vi "OEE_SCREEN_2.vi"(8 "error_in":errorcluster, 11 "all_config_info":T2={"main_ini_file"={"SQL Driver"="", "SQL Server"="", "SQL Database"="", "SQL UID"="", "Reference table"="", "Reference history"="", "Archivisation CFG table"="", "Archivisation CFG history"="", "User table"="", "User history"="", "Default reference"="", "Update pulse[ms]"=0, "default language"="", "SCREEN 1 Left"=0, "SCREEN 1 Top"=10, "SCREEN 1 Width"=0, "SCREEN 1 Height"=0, "SCREEN 2 Left"=0, "SCREEN 2 Top"=0, "SCREEN 2 Width"=0, "SCREEN 2 Height"=10}, "SQL Password"="", "queue_refnums"={"MAIN_queue"=refnum, "SCREEN_1_queue"=refnum, "SCREEN_2_queue"=refnum, "PULSE_queue"=refnum, "GRAPH_TOGGLE_queue"=refnum}}) -> (0 "error_out":errorcluster)   [LabVIEW 2020]
uses:
  ini/typedef/OEE_all_config_info.ctl
  ini/typedef/OEE_main_ini_file.ctl
  queues/typedef/OEE_queue_refnums.ctl
  queues/typedef/OEE_MAIN_queue_element.ctl
  MAIN/OEE_MAIN_sequence_state.ctl
  queues/typedef/OEE_SCREEN_1_queue_element.ctl
  SCREEN_1/OEE_SCREEN_1_sequence_state.ctl
  queues/typedef/OEE_SCREEN_2_queue_element.ctl
  OEE_SCREEN_2_sequence_state.ctl
  queues/typedef/OEE_PULSE_queue_element.ctl
  PULSE/OEE_PULSE_sequence_state.ctl
  queues/typedef/OEE_GRAPH_TOGGLE_TIMER_queue_element.ctl
  GRAPH_TOGGLE_TIMER/OEE_GRAPH_TOGGLE_TIMER_sequence_state.ctl
  typedef/SCREEN_2.ctl
  <vilib>/Utility/miscctls.llb/LVRectTypeDef.ctl
  FGV/FGV_SCREEN_2_graph_accumulative/FGV_SCREEN_2_graph_accumulative.ctl
  FGV/FGV_SCREEN_2_graph_accumulative/FGV_SCREEN_2_graph_accumulative_references.ctl
  FGV/FGV_SCREEN_2_graph_hourly/FGV_SCREEN_2_graph_hourly.ctl
  FGV/FGV_SCREEN_2_graph_hourly/FGV_SCREEN_2_graph_hourly_references.ctl
  <vilib>/Utility/error.llb/DialogType.ctl
  _misc/AULocalize/SubVIs/RegisterVI.vi
  _misc/AULocalize/SubVIs/Get Localized Phrase Compact Interface 0D.vi
panel:
  out "labels_picture_hourly":picture
  out "graph_hourly":cluster{dbl[], dbl[]}[](graph) caption="ПОЧАСОВАЯ ЦЕЛЬ VS АКТУАЛЬНЫЕ ЗНАЧЕНИЯ"
  out "labels_picture_accumulative":picture
  out "graph_accumulative":cluster{dbl[], dbl[]}[](graph) caption="НАКОПИТЕЛЬНАЯ ЦЕЛЬ VS АКТУАЛЬНЫЕ ЗНАЧЕНИЯ"
  out "SCREEN_2":T1={"header_part_no"="-", "header_customer"="-", "performance_percentage"="-", "performance_target"="-", "performance_actual"="-", "performance_header"="PERFORMANCE", "performance_target_header"="TARGET", "performance_actual_header"="ACTUAL", "screen_2_header"=""}
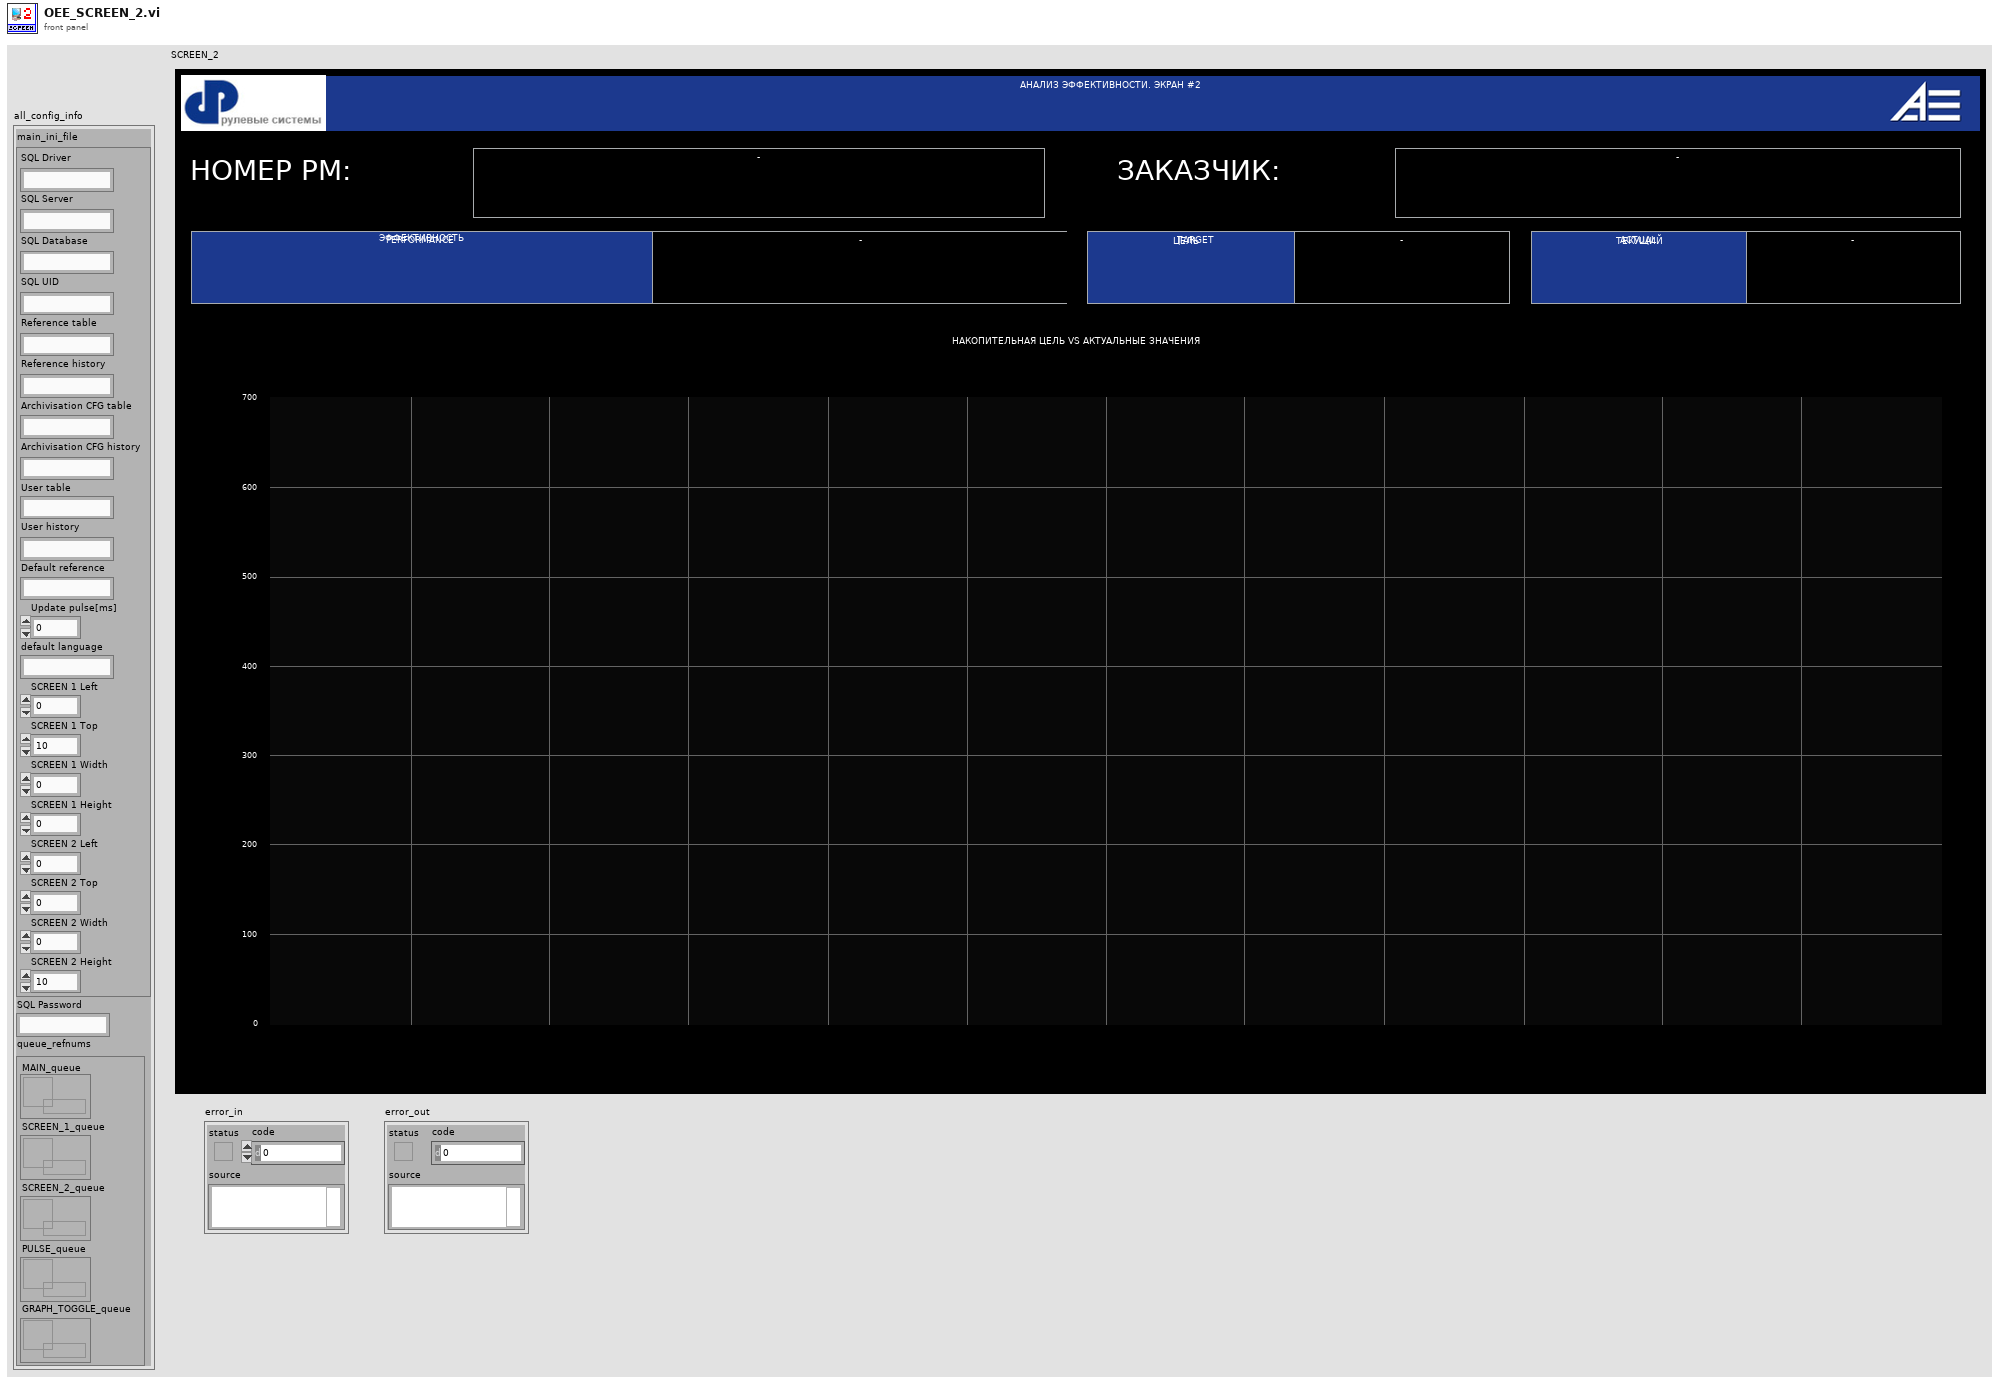
[diagram p1: front panel]
types:
  T1 = typedef "SCREEN_2.ctl" = cluster{"header_part_no":string, "header_customer":string, "performance_percentage":string, "performance_target":string, "performance_actual":string, "performance_header":string, "performance_target_header":string, "performance_actual_header":string, "screen_2_header":string}
  T2 = typedef "OEE_all_config_info.ctl" = cluster{"main_ini_file":T3, "SQL Password":string, "queue_refnums":T4}
  T3 = typedef "OEE_main_ini_file.ctl" = cluster{"SQL Driver":string, "SQL Server":string, "SQL Database":string, "SQL UID":string, "Reference table":string, "Reference history":string, "Archivisation CFG table":string, "Archivisation CFG history":string, "User table":string, "User history":string, "Default reference":string, "Update pulse[ms]":i32, "default language":string, "SCREEN 1 Left":i16, "SCREEN 1 Top":i16, "SCREEN 1 Width":i16, "SCREEN 1 Height":i16, "SCREEN 2 Left":i16, "SCREEN 2 Top":i16, "SCREEN 2 Width":i16, "SCREEN 2 Height":i16}
  T4 = typedef "OEE_queue_refnums.ctl" = cluster{"MAIN_queue":refnum<queue>, "SCREEN_1_queue":refnum<queue>, "SCREEN_2_queue":refnum<queue>, "PULSE_queue":refnum<queue>, "GRAPH_TOGGLE_queue":refnum<queue>}
  T5 = typedef "FGV_SCREEN_2_graph_hourly_references.ctl" = cluster{"graph_hourly":refnum<vi>, "labels_picture_hourly":refnum<vi>, "front_panel_reference":refnum<vi>}
  T6 = typedef "FGV_SCREEN_2_graph_hourly.ctl" = enum16{"initialize", "set_hour_start", "set_hour_end", "set_target", "set_actual", "toggle_visibility", "display"}
  T7 = typedef "FGV_SCREEN_2_graph_accumulative_references.ctl" = cluster{"graph_accumulative":refnum<vi>, "labels_picture_accumulative":refnum<vi>, "front_panel_reference":refnum<vi>}
  T8 = typedef "FGV_SCREEN_2_graph_accumulative.ctl" = enum16{"initialize", "set_hour_start", "set_hour_end", "set_target", "set_actual", "display"}
  T9 = typedef "LVRectTypeDef.ctl" = cluster{"Left":i16, "Top":i16, "Right":i16, "Bottom":i16}
  T10 = typedef "OEE_SCREEN_2_sequence_state.ctl" = enum16{"initialize", "get_next_state", "update", "show", "hide", "error", "stop"}
  T11 = typedef "OEE_GRAPH_TOGGLE_TIMER_sequence_state.ctl" = enum16{"initialize", "get_next_state", "start_toggling", "stop_toggling", "do_toggle", "error", "stop"}
  T12 = typedef "OEE_GRAPH_TOGGLE_TIMER_queue_element.ctl" = cluster{"state":T11, "variable":variant}
  T13 = typedef "OEE_SCREEN_2_queue_element.ctl" = cluster{"state":T10, "variable":variant}
  T14 = typedef "DialogType.ctl" = u16
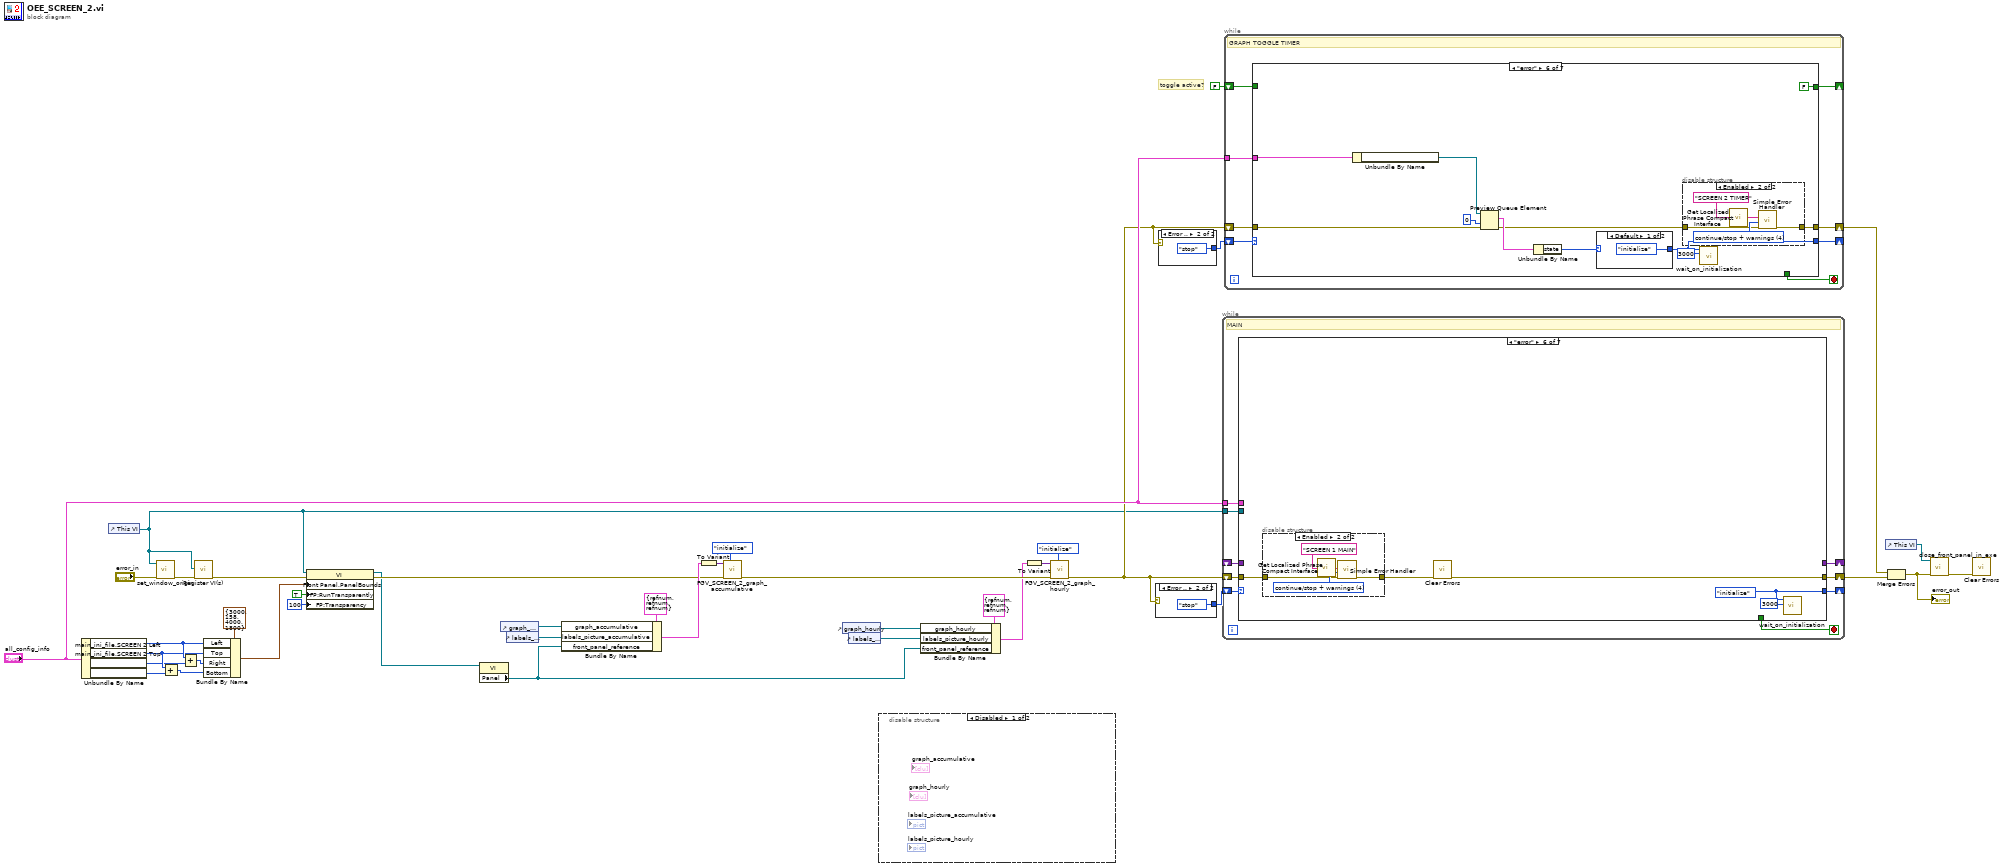
[diagram p0: block diagram]
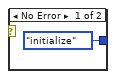
[diagram p2: hidden frame]
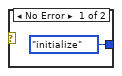
[diagram p3: hidden frame]
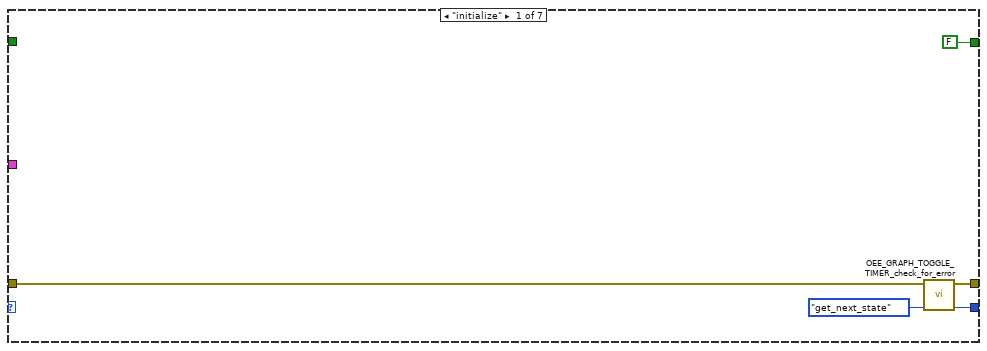
[diagram p4: hidden frame]
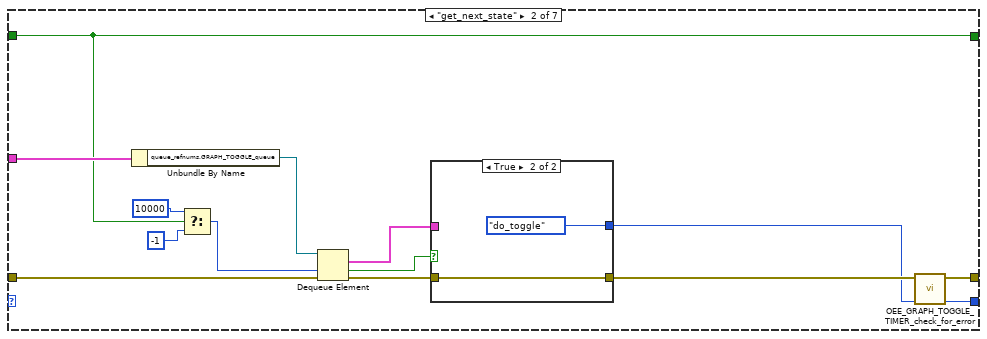
[diagram p5: hidden frame]
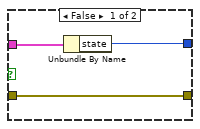
[diagram p6: hidden frame]
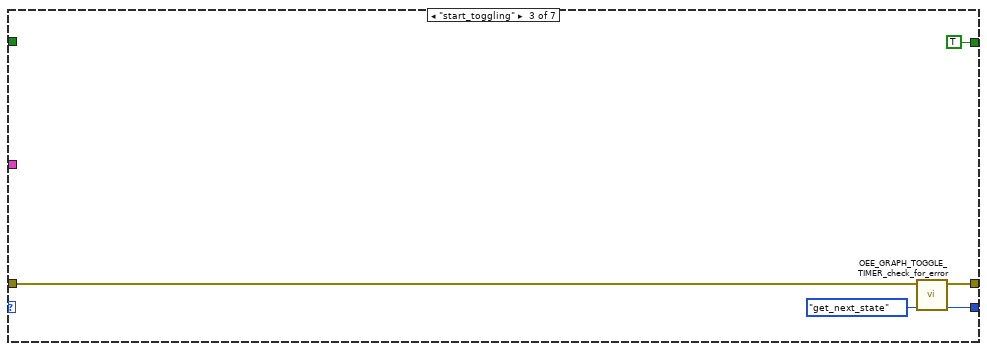
[diagram p7: hidden frame]
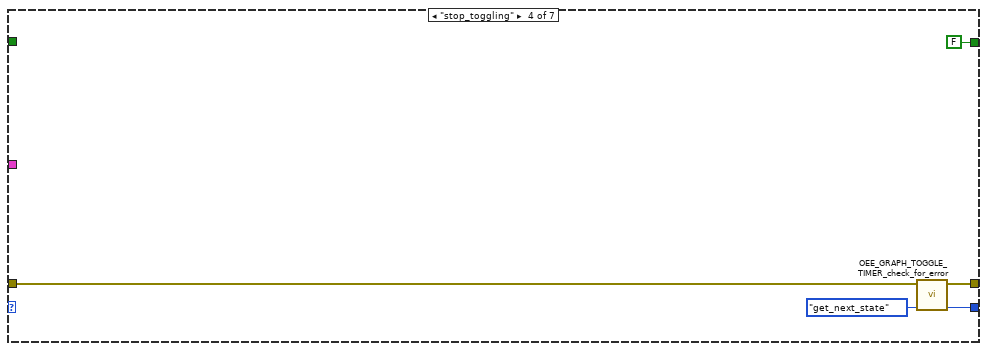
[diagram p8: hidden frame]
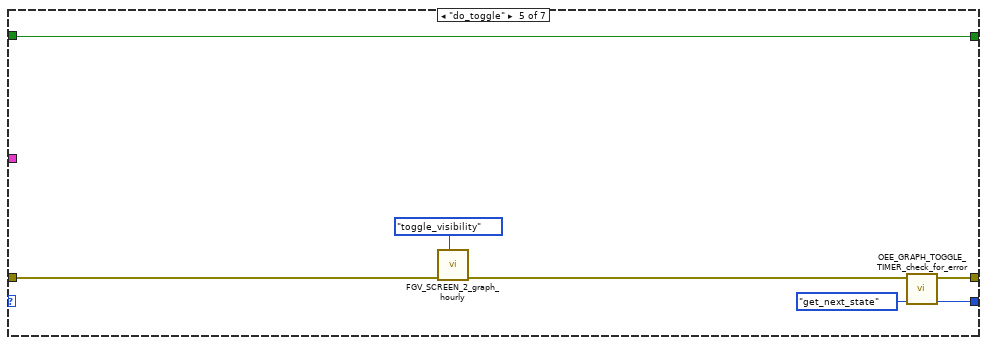
[diagram p9: hidden frame]
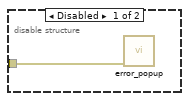
[diagram p10: hidden frame]
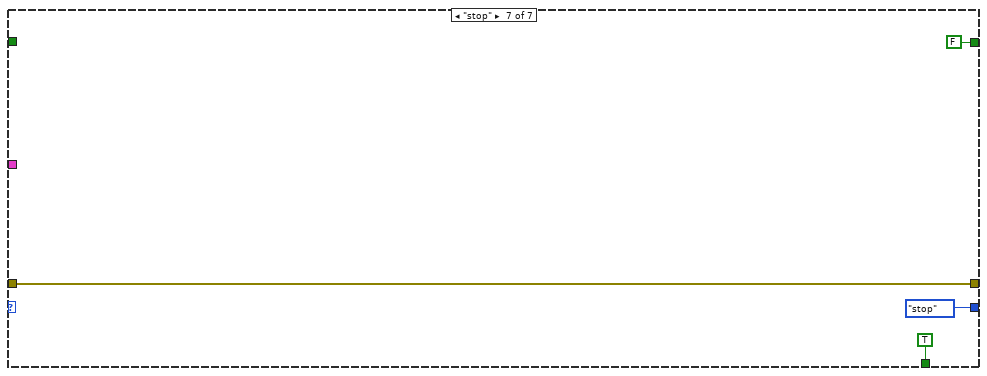
[diagram p12: hidden frame]
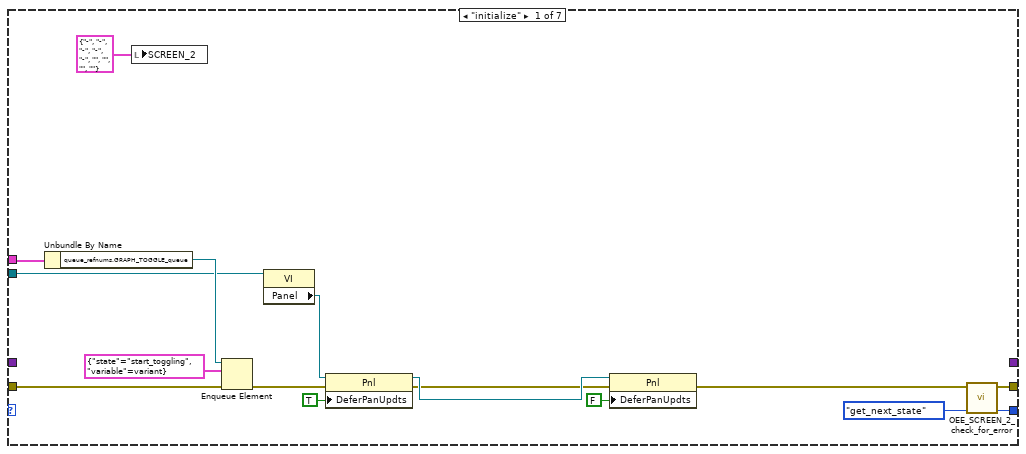
[diagram p14: hidden frame]
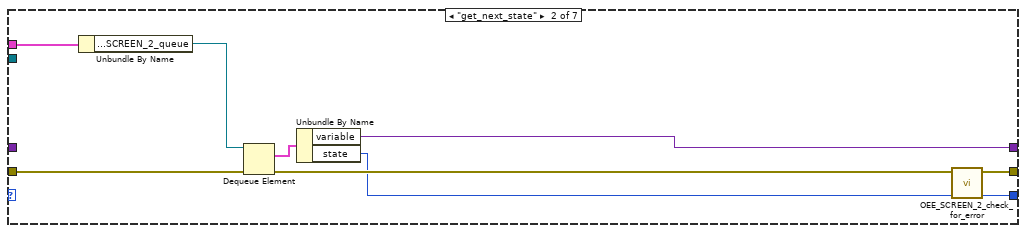
[diagram p15: hidden frame]
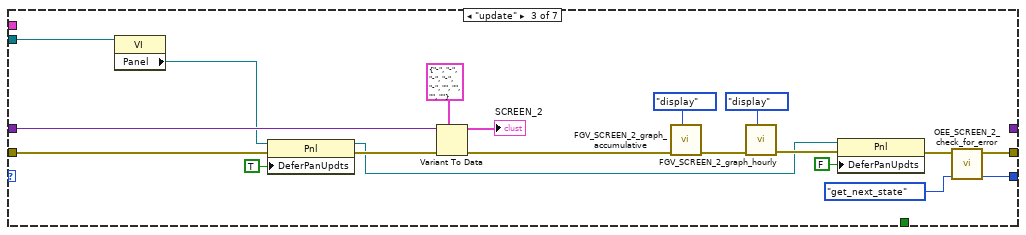
[diagram p16: hidden frame]
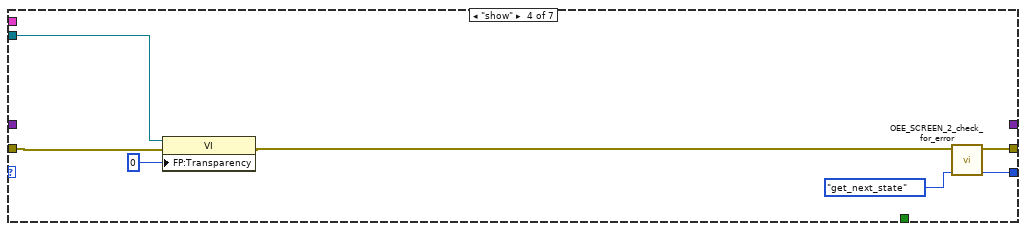
[diagram p17: hidden frame]
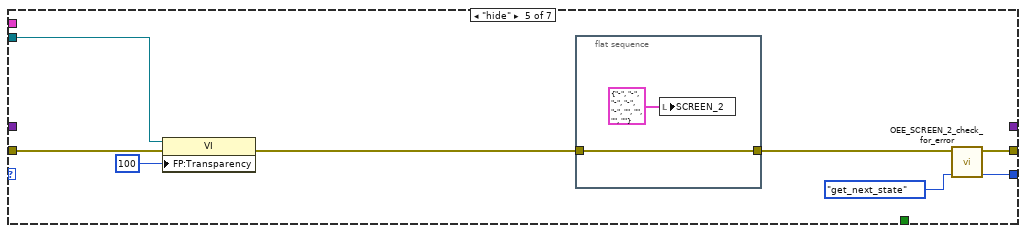
[diagram p18: hidden frame]
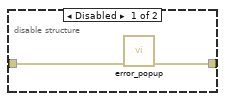
[diagram p19: hidden frame]
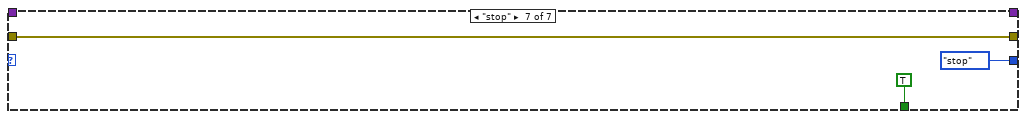
[diagram p20: hidden frame]
diagram:
  # "toggle active?"
  n1 = Unbundle By Name("all_config_info") -> ("main_ini_file.SCREEN 2 Left"=w36:i16, "main_ini_file.SCREEN 2 Top"=w35:i16, "main_ini_file.SCREEN 2 Width"=w34:i16, "main_ini_file.SCREEN 2 Height"=w33:i16)
  n2 = control-ref of="This VI"() -> (w1:refnum<vi>)
  n3 = call "set_window_origin.vi"("error_in"="error_in", "this_vi_reference"=w1) -> ("error_out"=w3:errorcluster)  [unwired: 9 in]
  n4 = Add(x=w35, y=w33) -> (x+y=w38:i16)
  n5 = Add(x=w36, y=w34) -> (x+y=w39:i16)
  n6 = call-poly "Register VI(s).vi"("error in"=w3, "VI Ref"=w1) -> ("error out"=w2:errorcluster)  [unwired: 8 in, 1 out]
  n7 = Bundle By Name(cluster=T9 {"Left"=3000, "Top"=158, "Right"=4000, "Bottom"=1800} ("Front Panel Window:Panel Bounds"), "Left"=w36, "Top"=w35, "Right"=w39, "Bottom"=w38) -> (w7:T9)
  n8 = property class="VI"(reference=w1, error in=w2, "Front Panel.PanelBounds"=w7, "FP:RunTransparently"=TRUE ("Front Panel Window:Run VI Transparently"), "FP:Transparency"=u8 100 ("Front Panel Window:Transparency")) -> (reference out=w8:refnum<vi>, error out=w9:errorcluster)
  n9 = property class="VI"(reference=w8) -> ("Panel"=w12:refnum<vi>)  [unwired: 1 in, 2 out]
  n10 = control-ref of="graph_accumulative"() -> (w30:refnum<vi>)
  n11 = control-ref of="labels_picture_accumulative"() -> (w19:refnum<vi>)
  n12 = Bundle By Name(cluster=T7 {"graph_accumulative"=refnum, "labels_picture_accumulative"=refnum, "front_panel_reference"=refnum} ("OBJ_references"), "graph_accumulative"=w30, "labels_picture_accumulative"=w19, "front_panel_reference"=w12) -> (w28:T7)
  n13 = To Variant(anything=w28) -> (Variant=w29:variant)
  n14 = call "FGV_SCREEN_2_graph_accumulative.vi"("options"=FGV_SCREEN_2_graph_accumulative."initialize", "error_in"=w9, "input"=w29) -> ("error_out"=w27:errorcluster)  [unwired: 8 in]
  n15 = control-ref of="graph_hourly"() -> (w22:refnum<vi>)
  n16 = control-ref of="labels_picture_hourly"() -> (w18:refnum<vi>)
  n17 = disable-structure shown="Disabled" {
    frame Disabled {
    }
    frame Enabled {
    }
  }
  n18 = Bundle By Name(cluster=T5 {"graph_hourly"=refnum, "labels_picture_hourly"=refnum, "front_panel_reference"=refnum} ("graph_hourly_references"), "graph_hourly"=w22, "labels_picture_hourly"=w18, "front_panel_reference"=w12) -> (w24:T5)
  n19 = To Variant(anything=w24) -> (Variant=w25:variant)
  n20 = call "FGV_SCREEN_2_graph_hourly.vi"("options"=FGV_SCREEN_2_graph_hourly."initialize", "error_in"=w27, "input"=w25) -> ("error_out"=w4:errorcluster)  [unwired: 8 in]
  n21 = case shown="Error .." w4 {
    tunnel: [OEE_SCREEN_2_sequence_state."initialize" ("state") OEE_SCREEN_2_sequence_state."stop" ("state")] -> w37
    frame No Error {
    }
    frame Error {
    }
  }
  n22 = case shown="Error .." w4 {
    tunnel: [OEE_GRAPH_TOGGLE_TIMER_sequence_state."initialize" ("OBJ_GUI_TIMER_sequence_state") OEE_GRAPH_TOGGLE_TIMER_sequence_state."stop" ("OBJ_GUI_TIMER_sequence_state")] -> w15
    frame No Error {
    }
    frame Error {
    }
  }
  n23 = while {
    shift-right: [w50] -> _
    shift-left: w37 -> [w51]
    shift-right: [w49] -> _
    shift-left: _ -> [w48]
    shift-right: [w52] -> w14
    shift-left: w4 -> [w53]
    tunnel: "all_config_info" -> [w46]
    tunnel: w1 -> [w45]
    stop <- w47 stop-if-true
    # "MAIN"
    n24 = case shown="\"error\"" w51 {
      tunnel: w53 -> [w65 w74 w82 w100 w108 w115 w129]
      tunnel: [w69 w78 w97 w104 w112 w119 w129] -> w52
      tunnel: [w68 w77 w96 w103 w111 w118 OEE_SCREEN_2_sequence_state."stop" ("state")] -> w50
      tunnel: [_ w72 _ _ _ _ _] -> w49
      tunnel: w48 -> [_ _ w89 _ _ _ _]
      tunnel: [_ _ _ _ _ _ TRUE] -> w47
      tunnel: w46 -> [w66 w71 _ _ _ _ _]
      tunnel: w45 -> [w56 _ w81 w99 w107 _ _]
      frame "initialize" {
        n25 = Unbundle By Name(w66) -> ("queue_refnums.GRAPH_TOGGLE_queue"=w64:refnum<queue>)
        n26 = local write "SCREEN_2"(T1 {"header_part_no"="-", "header_customer"="-", "performance_percentage"="-", "performance_target"="-", "performance_actual"="-", "performance_header"="", "performance_target_header"="", "performance_actual_header"="", "screen_2_header"=""} ("SCREEN_2")) -> ()
        n27 = Enqueue Element(queue=w64, element=T12 {"state"=enum."start_toggling", "variable"=variant}, error in (no error)=w65) -> (error out=w59:errorcluster)  [unwired: 1 in, 2 out]
        n28 = property class="VI"(reference=w56) -> ("Panel"=w55:refnum<vi>)  [unwired: 1 in, 2 out]
        n29 = property class="Pnl"(reference=w55, error in=w59, "DeferPanUpdts"=TRUE ("Defer Panel Updates")) -> (reference out=w57:refnum<vi>, error out=w54:errorcluster)
        n30 = property class="Pnl"(reference=w57, error in=w54, "DeferPanUpdts"=FALSE ("Defer Panel Updates")) -> (error out=w58:errorcluster)  [unwired: 1 out]
        n31 = call "OEE_SCREEN_2_check_for_error.vi"("SCREEN_2_loop_state_in"=OEE_SCREEN_2_sequence_state."get_next_state" ("state"), "error_in"=w58) -> ("SCREEN_2_loop_state_out"=w68:T10, "error_out"=w69:errorcluster)  [unwired: 8 in]
      }
      frame "get_next_state" {
        n32 = Unbundle By Name(w71) -> ("queue_refnums.SCREEN_2_queue"=w75:refnum<queue>)
        n33 = Dequeue Element(queue=w75, error in (no error)=w74) -> (element=w76:T13, error out=w73:errorcluster)  [unwired: 1 in, 2 out]
        n34 = Unbundle By Name(w76) -> ("variable"=w72:variant, "state"=w70:T10)
        n35 = call "OEE_SCREEN_2_check_for_error.vi"("SCREEN_2_loop_state_in"=w70, "error_in"=w73) -> ("SCREEN_2_loop_state_out"=w77:T10, "error_out"=w78:errorcluster)  [unwired: 8 in]
      }
      frame "update" {
        n36 = property class="VI"(reference=w81) -> ("Panel"=w80:refnum<vi>)  [unwired: 1 in, 2 out]
        n37 = property class="Pnl"(reference=w80, error in=w82, "DeferPanUpdts"=TRUE ("Defer Panel Updates")) -> (reference out=w85:refnum<vi>, error out=w92:errorcluster)
        n38 = Variant To Data(error in=w92, type=T1 {"header_part_no"="-", "header_customer"="-", "performance_percentage"="-", "performance_target"="-", "performance_actual"="-", "performance_header"="", "performance_target_header"="", "performance_actual_header"="", "screen_2_header"=""} ("SCREEN_2"), Variant=w89) -> (data=→"SCREEN_2":T1, error out=w79:errorcluster)
        n39 = call "FGV_SCREEN_2_graph_accumulative.vi"("options"=FGV_SCREEN_2_graph_accumulative."display", "error_in"=w79) -> ("error_out"=w93:errorcluster)  [unwired: 9 in]
        n40 = call "FGV_SCREEN_2_graph_hourly.vi"("options"=FGV_SCREEN_2_graph_hourly."display", "error_in"=w93) -> ("error_out"=w87:errorcluster)  [unwired: 9 in]
        n41 = property class="Pnl"(reference=w85, error in=w87, "DeferPanUpdts"=FALSE ("Defer Panel Updates")) -> (error out=w86:errorcluster)  [unwired: 1 out]
        n42 = call "OEE_SCREEN_2_check_for_error.vi"("SCREEN_2_loop_state_in"=OEE_SCREEN_2_sequence_state."get_next_state", "error_in"=w86) -> ("SCREEN_2_loop_state_out"=w96:T10, "error_out"=w97:errorcluster)  [unwired: 8 in]
      }
      frame "show" {
        n43 = property class="VI"(reference=w99, error in=w100, "FP:Transparency"=u8 0 ("Front Panel Window:Transparency")) -> (error out=w98:errorcluster)  [unwired: 1 out]
        n44 = call "OEE_SCREEN_2_check_for_error.vi"("SCREEN_2_loop_state_in"=OEE_SCREEN_2_sequence_state."get_next_state", "error_in"=w98) -> ("SCREEN_2_loop_state_out"=w103:T10, "error_out"=w104:errorcluster)  [unwired: 8 in]
      }
      frame "hide" {
        n45 = property class="VI"(reference=w107, error in=w108, "FP:Transparency"=u8 100 ("Front Panel Window:Transparency")) -> (error out=w105:errorcluster)  [unwired: 1 out]
        n46 = flat-sequence {
          tunnel: w105 -> [w113]
          tunnel: [w113] -> w106
          frame #0 {
            n47 = local write "SCREEN_2"(T1 {"header_part_no"="-", "header_customer"="-", "performance_percentage"="-", "performance_target"="-", "performance_actual"="-", "performance_header"="", "performance_target_header"="", "performance_actual_header"="", "screen_2_header"=""} ("SCREEN_2")) -> ()
          }
        }
        n48 = call "OEE_SCREEN_2_check_for_error.vi"("SCREEN_2_loop_state_in"=OEE_SCREEN_2_sequence_state."get_next_state", "error_in"=w106) -> ("SCREEN_2_loop_state_out"=w111:T10, "error_out"=w112:errorcluster)  [unwired: 8 in]
      }
      frame "error" {
        w118 = OEE_SCREEN_2_sequence_state."initialize" ("state")
        n49 = disable-structure shown="Enabled" {
          disable-tunnel: w115 -> [w121 w123]
          disable-tunnel: [w120 w126] -> w116
          frame Disabled {
            n50 = call "error_popup.vi"("error_in"=w121) -> ("error_out"=w120:errorcluster)  [unwired: 10 in]
          }
          frame Enabled {
            w124 = T14 4 items=["no dialog", "OK message", "continue or stop message", "OK message + warnings", "continue/stop + warnings"] ("type of dialog (OK msg:1)")
            n51 = call-poly "Get Localized Phrase Compact Interface.vi"("Key"="SCREEN 1 MAIN" ("error source (\" \")")) -> ("Translated Phrase"=w122:string)
            n52 = call <vilib>:"Simple Error Handler.vi"("error source (\" \")"=w122, "type of dialog (OK msg:1)"=w124, "error in (no error)"=w123) -> ("error out"=w126:errorcluster)  [unwired: 2 in, 4 out]
          }
        }
        n53 = call <vilib>:"Clear Errors.vi"("error in (no error)"=w116) -> ("error out"=w119:errorcluster)  [unwired: 5 in, 1 out]
        n54 = call "wait_on_initialization.vi"("milliseconds_to_wait(1000)"=u32 3000, "state"=w118) -> ()  [unwired: 10 in]
      }
      frame "stop" {
      }
    }
  }
  n55 = while {
    tunnel: "all_config_info" -> [w137]
    shift-right: [w134] -> _
    shift-left: w15 -> [w136]
    shift-right: [w133] -> w13
    shift-left: w4 -> [w135]
    shift-right: [w132] -> _
    shift-left: FALSE -> [w131]
    stop <- w130 stop-if-true
    # "GRAPH TOGGLE TIMER"
    n56 = case shown="\"error\"" w136 {
      tunnel: w137 -> [_ w155 _ _ _ w185 _]
      tunnel: w135 -> [w142 w154 w162 w167 w174 w182 w199]
      tunnel: [w140 w147 w164 w169 w177 w184 OEE_GRAPH_TOGGLE_TIMER_sequence_state."stop" ("OBJ_GUI_TIMER_sequence_state")] -> w134
      tunnel: [w141 w148 w165 w170 w178 w179 w199] -> w133
      tunnel: [FALSE w153 TRUE FALSE w175 FALSE FALSE] -> w132
      tunnel: w131 -> [_ w153 _ _ w175 _ _]
      tunnel: [_ _ _ _ _ _ TRUE] -> w130
      frame "initialize" {
        n57 = call "OEE_GRAPH_TOGGLE_TIMER_check_for_error.vi"("GRAPH_TOGGLE_TIMER_loop_state_in"=OEE_GRAPH_TOGGLE_TIMER_sequence_state."get_next_state" ("GUI_TIMER_loop_state_in"), "error_in"=w142) -> ("GRAPH_TOGGLE_TIMER_loop_state_out"=w140:T11, "error_out"=w141:errorcluster)  [unwired: 8 in]
      }
      frame "get_next_state" {
        n58 = Unbundle By Name(w155) -> ("queue_refnums.GRAPH_TOGGLE_queue"=w156:refnum<queue>)
        n59 = Select(t=10000, s=w153, f=-1 ("timeout in ms (-1)")) -> (s? t:f=w150:i32)
        n60 = Dequeue Element(queue=w156, timeout in ms (-1)=w150, error in (no error)=w154) -> (element=w145:T12, timed out?=w149:bool, error out=w146:errorcluster)  [unwired: 1 out]
        n61 = case shown="True" w149 {
          tunnel: w146 -> [w159 w161]
          tunnel: w145 -> [w158 _]
          tunnel: [w159 w161] -> w144
          tunnel: [w157 OEE_GRAPH_TOGGLE_TIMER_sequence_state."do_toggle" ("state")] -> w143
          frame False {
            n62 = Unbundle By Name(w158) -> ("state"=w157:T11)
          }
          frame True {
          }
        }
        n63 = call "OEE_GRAPH_TOGGLE_TIMER_check_for_error.vi"("GRAPH_TOGGLE_TIMER_loop_state_in"=w143, "error_in"=w144) -> ("GRAPH_TOGGLE_TIMER_loop_state_out"=w147:T11, "error_out"=w148:errorcluster)  [unwired: 8 in]
      }
      frame "start_toggling" {
        n64 = call "OEE_GRAPH_TOGGLE_TIMER_check_for_error.vi"("GRAPH_TOGGLE_TIMER_loop_state_in"=OEE_GRAPH_TOGGLE_TIMER_sequence_state."get_next_state" ("GUI_TIMER_loop_state_in"), "error_in"=w162) -> ("GRAPH_TOGGLE_TIMER_loop_state_out"=w164:T11, "error_out"=w165:errorcluster)  [unwired: 8 in]
      }
      frame "stop_toggling" {
        n65 = call "OEE_GRAPH_TOGGLE_TIMER_check_for_error.vi"("GRAPH_TOGGLE_TIMER_loop_state_in"=OEE_GRAPH_TOGGLE_TIMER_sequence_state."get_next_state" ("GUI_TIMER_loop_state_in"), "error_in"=w167) -> ("GRAPH_TOGGLE_TIMER_loop_state_out"=w169:T11, "error_out"=w170:errorcluster)  [unwired: 8 in]
      }
      frame "do_toggle" {
        n66 = call "FGV_SCREEN_2_graph_hourly.vi"("options"=FGV_SCREEN_2_graph_hourly."toggle_visibility", "error_in"=w174) -> ("error_out"=w173:errorcluster)  [unwired: 9 in]
        n67 = call "OEE_GRAPH_TOGGLE_TIMER_check_for_error.vi"("GRAPH_TOGGLE_TIMER_loop_state_in"=OEE_GRAPH_TOGGLE_TIMER_sequence_state."get_next_state" ("GUI_TIMER_loop_state_in"), "error_in"=w173) -> ("GRAPH_TOGGLE_TIMER_loop_state_out"=w177:T11, "error_out"=w178:errorcluster)  [unwired: 8 in]
      }
      frame "error" {
        n68 = Unbundle By Name(w185) -> ("queue_refnums.GRAPH_TOGGLE_queue"=w189:refnum<queue>)
        n69 = Preview Queue Element(queue=w189, timeout in ms (-1)=0, error in (no error)=w182) -> (element=w187:T12, error out=w180:errorcluster)  [unwired: 2 out]
        n70 = Unbundle By Name(w187) -> ("state"=w188:T11)
        n71 = case shown="Default" w188 {
          selector: w188 -> [_ w198]
          tunnel: [OEE_GRAPH_TOGGLE_TIMER_sequence_state."initialize" ("OBJ_GUI_TIMER_sequence_state") w198] -> w184
          frame Default {
          }
          frame "stop" {
          }
        }
        n72 = disable-structure shown="Enabled" {
          disable-tunnel: w180 -> [w191 w194]
          disable-tunnel: [_ w193] -> w179
          frame Disabled {
            n73 = call "error_popup.vi"("error_in"=w191) -> ("error_out"=w190:errorcluster)  [unwired: 10 in]
          }
          frame Enabled {
            w195 = T14 4 items=["no dialog", "OK message", "continue or stop message", "OK message + warnings", "continue/stop + warnings"] ("type of dialog (OK msg:1)")
            n74 = call-poly "Get Localized Phrase Compact Interface.vi"("Key"="SCREEN 2 TIMER" ("error source (\" \")")) -> ("Translated Phrase"=w192:string)
            n75 = call <vilib>:"Simple Error Handler.vi"("error source (\" \")"=w192, "type of dialog (OK msg:1)"=w195, "error in (no error)"=w194) -> ("error out"=w193:errorcluster)  [unwired: 2 in, 4 out]
          }
        }
        n76 = call "wait_on_initialization.vi"("milliseconds_to_wait(1000)"=u32 3000, "state"=w184) -> ()  [unwired: 10 in]
      }
      frame "stop" {
      }
    }
  }
  n77 = control-ref of="This VI"() -> (w21:refnum<vi>)
  n78 = Merge Errors(w13, w14) -> (w5:errorcluster)
  "error_out" <- w5
  n79 = call "close_front_panel_in_exe.vi"("error_in"=w5, "vi_reference_in"=w21) -> ("error_out"=w20:errorcluster)  [unwired: 9 in]
  n80 = call <vilib>:"Clear Errors.vi"("error in (no error)"=w20) -> ()  [unwired: 5 in, 2 out]
